vi "Edge Detect.vi"(1 "State":bool=TRUE) -> (0 "Changed?":bool)   [LabVIEW 2011]
panel:
  in  "PreviousState":bool=TRUE
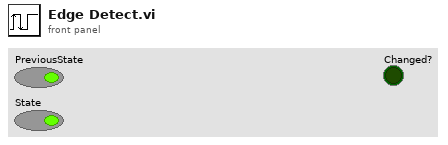
[diagram p1: front panel]
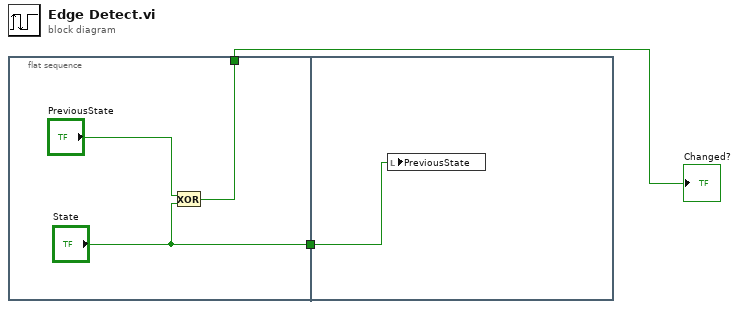
[diagram p0: block diagram]
diagram:
  n1 = flat-sequence {
    tunnel: ["State"] -> w2
    tunnel: [w3] -> w1
    tunnel: w2 -> [w6]
    frame #0 {
      n2 = Exclusive Or(1:"State", 2:"PreviousState") -> (0:w3:bool)
    }
    frame #1 {
      n3 = local write "PreviousState"(w6) -> ()
    }
  }
  "Changed?" <- w1
